vi "写入功率控制表.vi"(6 "预备区功率":string, 7 "Table输入":refnum<vi>, 8 "偏置2":u16, 9 "偏置1":u16, 10 "衰减器2":u16, 11 "衰减器1":u16) -> ()   [LabVIEW 2015]
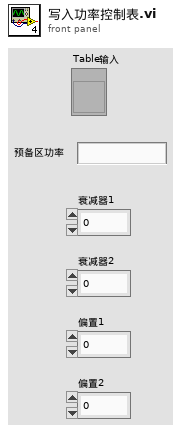
[diagram p1: front panel]
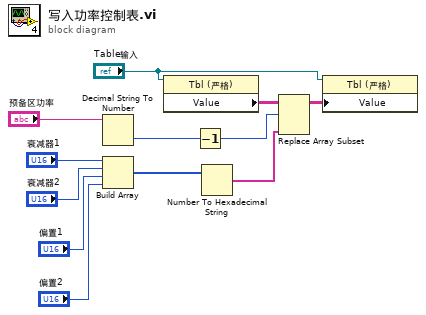
[diagram p0: block diagram]
diagram:
  n1 = Decimal String To Number(string="预备区功率") -> (number=w2:i32)  [unwired: 2 in, 1 out]
  n2 = Build Array("衰减器1", "衰减器2", "偏置1", "偏置2") -> (w7:u16[])
  n3 = property class="Tbl (严格)"(reference="Table输入") -> ("Value"=w8:string[][])  [unwired: 1 in, 2 out]
  n4 = Decrement(x=w2) -> (x-1=w9:i32)
  n5 = Number To Hexadecimal String(2:w7) -> (0:w10:string[])  [unwired: 1 in]
  n6 = Replace Array Subset(array=w8, new element=w10, index (row)=w9) -> (w11:string[][])  [unwired: 1 in]
  n7 = property class="Tbl (严格)"(reference="Table输入", "Value"=w11) -> ()  [unwired: 1 in, 2 out]
